vi "Dual Camera Control.vi"(7 "Calling VI Ref":refnum<vi>) -> ()   [LabVIEW 2016]
uses:
  Dual Camera Controls/Dual Camera - Simple Control.ctl
  <vilib>/Utility/miscctls.llb/LVPointTypeDef.ctl
  Hardware Configuration/Hardware Configuration Controls/Device Type.ctl
  Hardware Configuration/Hardware Configuration Controls/Device Function.ctl
  Device Library/Cameras/Photometrics/Prime BSI/Prime BSI Controls/Prime Actions.ctl
  Device Library/AOTF and AOM/AOTF Controls/AOTF Actions.ctl
  Device Library/Cameras/Photometrics/Prime BSI/Prime BSI Controls/Prime Parameters.ctl
  Device Library/Cameras/Photometrics/Prime BSI/Prime BSI Controls/Prime Parameter List.ctl
  Device Library/Stages/Stages Controls/Stage Actions.ctl
  Device Library/Cameras/Photometrics/Prime BSI/Prime BSI Controls/Prime ROI.ctl
  <vilib>/vision/Image Controls.llb/IMAQ Image.ctl
panel:
  in  "WFDC Z Step":bool
  in  "No. of Steps":i32
  in  "Step Size (µm)":dbl
  in  "Z Stack":bool
  in  "Cycles":u32
  in  "Delay Time (s)":u32
  in  "Delay Capture":bool
  in  "Both Cameras":T1 {"Exposure Time (s)" format="%#_4g"}
  in  "Camera 02":T1 {"Exposure Time (s)" format="%#_4g"}
  in  "Camera 01":T1 {"Exposure Time (s)" format="%#_4g"}
  in  "Quit":bool
  # "Camera 01"
  # "Camera 02"
  # "Both Cams"
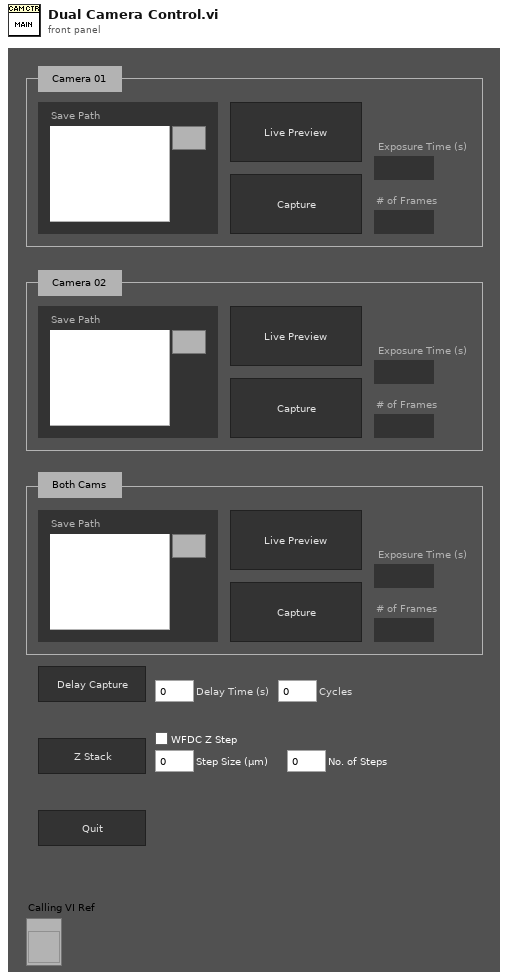
[diagram p1: front panel]
types:
  T1 = typedef "Dual Camera - Simple Control.ctl" = cluster{"Save Path":path, "Live Preview":bool, "Capture":bool, "Exposure Time (s)":dbl, "# of Frames":u32}
  T2 = enum16{"Always On", "Always Off", "Off While Running"}
  T3 = typedef "LVPointTypeDef.ctl" = cluster{"Horizontal":i16, "Vertical":i16}
  T4 = typedef "Device Function.ctl" = enum16{"Primary", "Secondary", "Overview", "Wide Field Drift Correction", "642 nm Excitation", "560 nm Excitation", "546 nm Excitation", "488 nm Excitation", "405 nm Excitation", "Objective Drift Correction", "Objective XY", "Objective Z", "Sample XY", "Sample Coarse Z", "Sample Z", "4Pi Lower", "4Pi Upper", "Adj Cavity", "Line Scanning", "Alert"}
  T5 = typedef "Device Type.ctl" = enum16{"AOTF", "Camera", "Deformable Mirror", "Laser", "Shutter", "Stage", "Waveform", "Email"}
  T6 = typedef "IMAQ Image.ctl" = refnum<image>
  T7 = typedef "Prime ROI.ctl" = cluster{"X Start":u32, "X End":u32, "X Bin":u32, "Y Start":u32, "Y End":u32, "Y Bin":u32}
  T8 = typedef "Prime Parameters.ctl" = cluster{"Parameter":T9, "Value":dbl}
  T9 = typedef "Prime Parameter List.ctl" = enum16{"Exposure Time (s)"}
  T10 = typedef "Prime Actions.ctl" = enum16{"Error Check", "Initialize", "Preview", "Record", "Abort", "Record Settings", "Set Parameter", "Get Parameter", "Set ROI", "Get ROI", "Status", "Set Trigger", "Quit"}
  T11 = typedef "AOTF Actions.ctl" = enum16{"Error Check", "Blank", "Line On/Off", "Set Power", "Status", "Quit"}
  T12 = typedef "Stage Actions.ctl" = enum16{"Get Position", "MVR", "MOVE", "HALT", "ONTARGET", "ERROR", "REFERENCE", "INIT", "VELOCITY", "STATUS", "EXIT", "HOME", "ZEROPOS", "NANOPOS", "ANALOG", "QUIT"}
  T13 = enum8{"Enabled", "Disabled", "Disabled and Grayed Out"}
  T14 = cluster{"Save Path":bool, "Live Preview":bool, "Capture":bool, "Exposure Time (s)":bool, "# of Frames":bool}
  T15 = typedef "LVRectTypeDef.ctl" = cluster{"Left":i16, "Top":i16, "Right":i16, "Bottom":i16}
  T16 = typedef "LVBoundsTypeDef.ctl" = cluster{"Width":u32, "Height":u32}
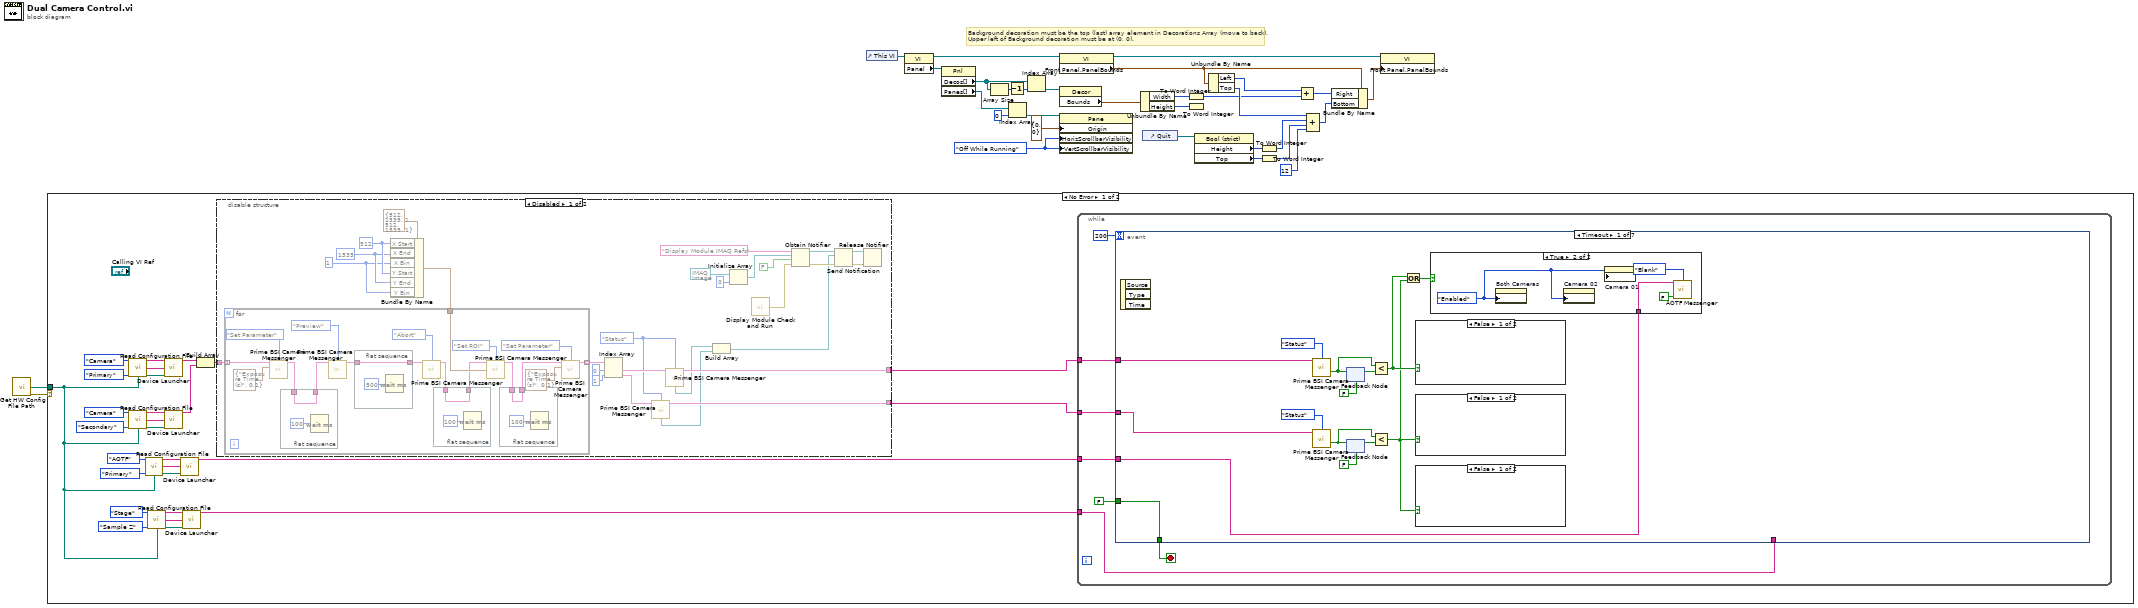
[diagram p0: block diagram]
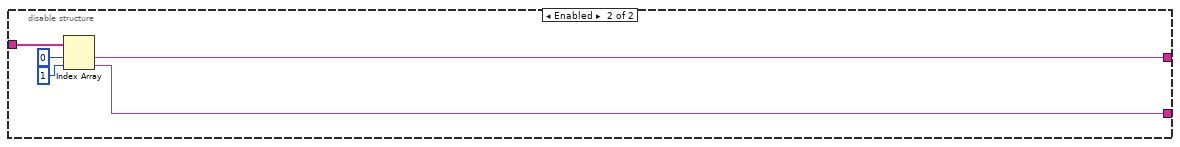
[diagram p2: hidden frame]
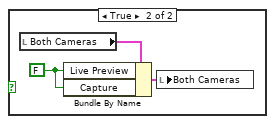
[diagram p4: hidden frame]
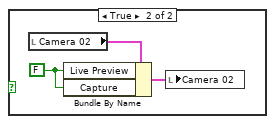
[diagram p5: hidden frame]
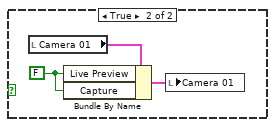
[diagram p6: hidden frame]
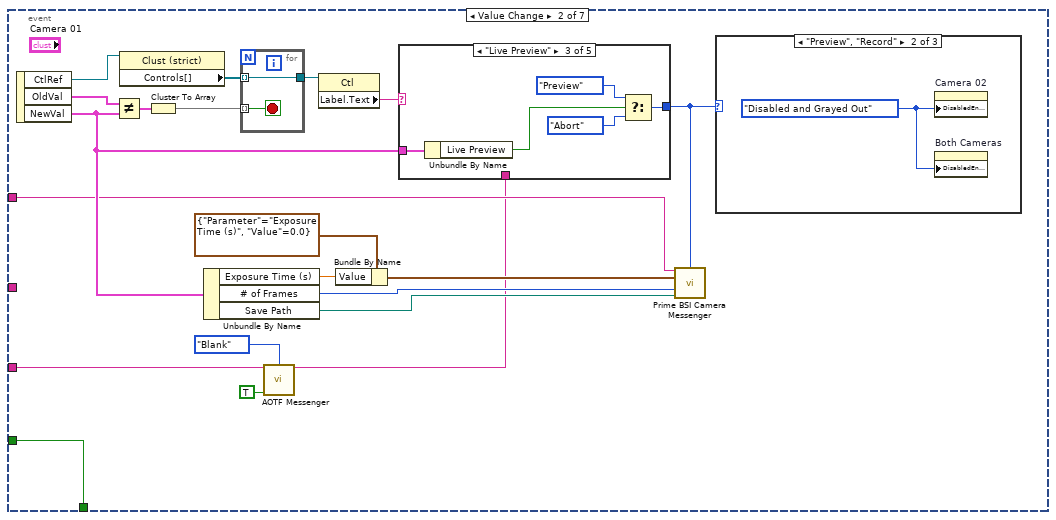
[diagram p7: hidden frame]
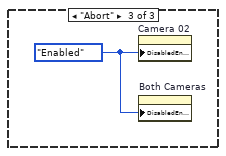
[diagram p9: hidden frame]
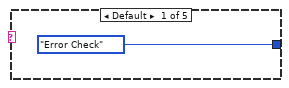
[diagram p10: hidden frame]
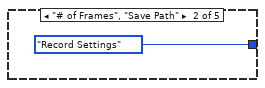
[diagram p11: hidden frame]
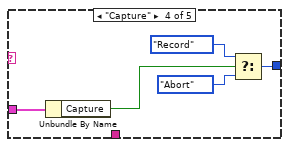
[diagram p12: hidden frame]
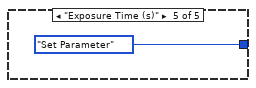
[diagram p13: hidden frame]
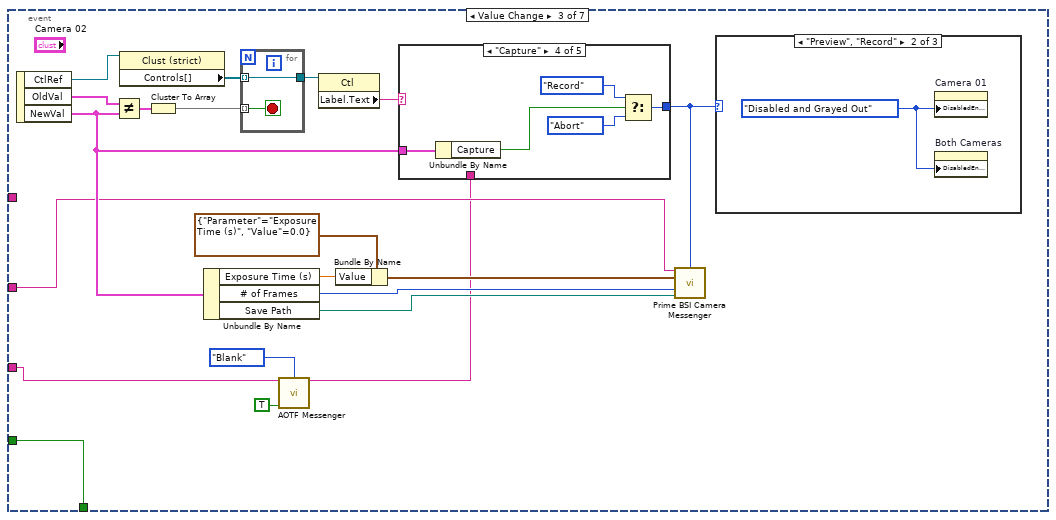
[diagram p14: hidden frame]
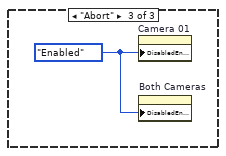
[diagram p16: hidden frame]
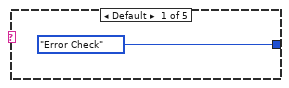
[diagram p17: hidden frame]
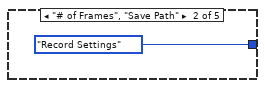
[diagram p18: hidden frame]
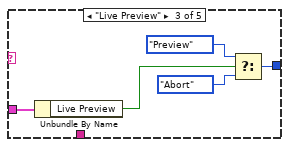
[diagram p19: hidden frame]
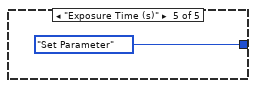
[diagram p20: hidden frame]
diagram:
  w14 = T2."Off While Running" ("Vertical Scrollbar Visibility")
  # "Background decoration must be the top (last) array element in Decorations Array (move to back).\nUpper left of Background decoration must be at (0, 0)."
  n1 = call "Get HW Config File Path.vi"() -> ("File Path"=w1:path, "Error"=w2:errorcluster)  [unwired: 14 in]
  n2 = case shown="No Error" w2 {
    tunnel: w1 -> [w38 _]
    frame No Error {
      n3 = call "Read Configuration File.vi"("Device Type"=Device_Type."Camera", "Device Function"=Device_Function."Primary", "Config File Path"=w38) -> ("Unique Notifier Name"=w59:string, "Device Ports/IDs/Channels"=w57:string[], "Device Engine Path"=w58:path)  [unwired: 9 in, 1 out]
      n4 = call "Read Configuration File.vi"("Device Type"=Device_Type."Camera", "Device Function"=Device_Function."Secondary", "Config File Path"=w38) -> ("Unique Notifier Name"=w50:string, "Device Ports/IDs/Channels"=w52:string[], "Device Engine Path"=w51:path)  [unwired: 9 in, 1 out]
      n5 = call "Read Configuration File.vi"("Device Type"=Device_Type."AOTF", "Device Function"=Device_Function."Primary", "Config File Path"=w38) -> ("Unique Notifier Name"=w49:string, "Device Ports/IDs/Channels"=w47:string[], "Device Engine Path"=w48:path)  [unwired: 9 in, 1 out]
      n6 = call "Read Configuration File.vi"("Device Type"=Device_Type."Stage", "Device Function"=Device_Function."Sample Z", "Config File Path"=w38) -> ("Unique Notifier Name"=w39:string, "Device Ports/IDs/Channels"=w41:string[], "Device Engine Path"=w40:path)  [unwired: 9 in, 1 out]
      n7 = call "Device Launcher.vi"("Notifier Name"=w59, "Device Ports/IDs/Channels"=w57, "Device Engine Path"=w58) -> ("Notifier Name"=w36:string)  [unwired: 11 in, 1 out]
      n8 = call "Device Launcher.vi"("Notifier Name"=w50, "Device Ports/IDs/Channels"=w52, "Device Engine Path"=w51) -> ("Notifier Name"=w35:string)  [unwired: 11 in, 1 out]
      n9 = call "Device Launcher.vi"("Notifier Name"=w49, "Device Ports/IDs/Channels"=w47, "Device Engine Path"=w48) -> ("Notifier Name"=w44:string)  [unwired: 11 in, 1 out]
      n10 = call "Device Launcher.vi"("Notifier Name"=w39, "Device Ports/IDs/Channels"=w41, "Device Engine Path"=w40) -> ("Notifier Name"=w37:string)  [unwired: 11 in, 1 out]
      n11 = Build Array(w36, w35) -> (w34:string[])
      n12 = disable-structure shown="Disabled" {
        disable-tunnel: w34 -> [w86 w115]
        disable-tunnel: [w76 w114] -> w33
        disable-tunnel: [w74 w113] -> w32
        frame Disabled {
          w75 = Prime_Actions."Status" ("Prime Actions")
          w79 = u32 1 ("X Bin")
          w80 = u32 1535 ("X End")
          w81 = u32 512 ("X Start")
          n13 = Bundle By Name(cluster=T7 {"X Start"=512, "X End"=1535, "X Bin"=1, "Y Start"=512, "Y End"=1535, "Y Bin"=1} ("ROI Setup"), "X Start"=w81, "X End"=w80, "X Bin"=w79, "Y Start"=w81, "Y End"=w80, "Y Bin"=w79) -> (w78:T7)
          n14 = for {
            tunnel: w86 -> [w95] mode=indexing
            tunnel: [w94] -> w85 mode=indexing
            tunnel: w78 -> [w93]
            n15 = call "Prime BSI Camera Messenger.vi"("Notifier Name"=w95, "Prime Actions"=Prime_Actions."Set Parameter", "Prime Parameter"=T8 {"Parameter"=enum."Exposure Time (s)", "Value"=0.1}) -> ("Notifier Name (Dup)"=w92:string)  [unwired: 7 in, 5 out]
            n16 = flat-sequence {
              tunnel: [w109] -> w91
              tunnel: w92 -> [w109]
              frame #0 {
                n17 = Wait (ms)(milliseconds to wait=u32 100) -> ()  [unwired: 1 out]
              }
            }
            n18 = call "Prime BSI Camera Messenger.vi"("Notifier Name"=w91, "Prime Actions"=Prime_Actions."Preview") -> ("Notifier Name (Dup)"=w102:string)  [unwired: 8 in, 5 out]
            n19 = flat-sequence {
              tunnel: w102 -> [w112]
              tunnel: [w112] -> w99
              frame #0 {
                n20 = Wait (ms)(milliseconds to wait=u32 500) -> ()  [unwired: 1 out]
              }
            }
            n21 = call "Prime BSI Camera Messenger.vi"("Notifier Name"=w99, "Prime Actions"=Prime_Actions."Abort") -> ("Notifier Name (Dup)"=w90:string)  [unwired: 8 in, 5 out]
            n22 = flat-sequence {
              tunnel: [w107] -> w89
              tunnel: w90 -> [w107]
              frame #0 {
                n23 = Wait (ms)(milliseconds to wait=u32 100) -> ()  [unwired: 1 out]
              }
            }
            n24 = call "Prime BSI Camera Messenger.vi"("Notifier Name"=w89, "Prime Actions"=Prime_Actions."Set ROI", "ROI Setup"=w93) -> ("Notifier Name (Dup)"=w88:string)  [unwired: 7 in, 5 out]
            n25 = flat-sequence {
              tunnel: [w105] -> w87
              tunnel: w88 -> [w105]
              frame #0 {
                n26 = Wait (ms)(milliseconds to wait=u32 100) -> ()  [unwired: 1 out]
              }
            }
            n27 = call "Prime BSI Camera Messenger.vi"("Notifier Name"=w87, "Prime Actions"=Prime_Actions."Set Parameter", "Prime Parameter"=T8 {"Parameter"=enum."Exposure Time (s)", "Value"=0.1}) -> ("Notifier Name (Dup)"=w94:string)  [unwired: 7 in, 5 out]
          }
          n28 = Index Array(array=w85, index #1=0 ("index"), index #2=1 ("index")) -> (element #1=w77:string, element #2=w60:string)
          n29 = call "Prime BSI Camera Messenger.vi"("Notifier Name"=w60, "Prime Actions"=w75) -> ("Notifier Name (Dup)"=w74:string, "Image Ref"=w72:T6)  [unwired: 8 in, 4 out]
          n30 = call "Prime BSI Camera Messenger.vi"("Notifier Name"=w77, "Prime Actions"=w75) -> ("Notifier Name (Dup)"=w76:string, "Image Ref"=w73:T6)  [unwired: 8 in, 4 out]
          n31 = Build Array(w73, w72) -> (w61:T6[])
          n32 = Initialize Array(T6 refnum ("New Image"), 0 ("dimension size")) -> (w70:T6[])
          n33 = call "Display Module Check and Run.vi"() -> ("Error"=w71:errorcluster)  [unwired: 15 in]
          n34 = Obtain Notifier(name (unnamed)="Display Module IMAQ Refs", notification data type=w70, create if not found? (T)=FALSE, error in (no error)=w71) -> (notifier out=w62:refnum<notifier>, error out=w65:errorcluster)  [unwired: 1 out]
          n35 = Send Notification(notification=w61, notifier=w62, error in (no error)=w65) -> (notifier out=w63:refnum<notifier>, error out=w64:errorcluster)
          n36 = Release Notifier(notifier=w63, error in (no error)=w64) -> ()  [unwired: 1 in, 3 out]
        }
        frame Enabled {
          n37 = Index Array(array=w115, index #1=0 ("index"), index #2=1 ("index")) -> (element #1=w114:string, element #2=w113:string)
        }
      }
      n38 = while {
        tunnel: w33 -> [w121]
        tunnel: w32 -> [w120]
        tunnel: w44 -> [w119]
        tunnel: w37 -> [w118]
        stop <- w123 stop-if-true
        n39 = event shown="[0] Timeout" {
          selector: _ -> [_ _ _ _ _ _ _]
          dyn-events: _ -> [_ _ _ _ _ _ _]
          timeout: 200 -> [_ _ _ _ _ _ _]
          tunnel: [w139 w172 w209 w255 w277 w349 w408] -> w123
          tunnel: FALSE -> [w139 w172 w209 w255 w277 w349 _]
          tunnel: w121 -> [w138 w158 _ w244 w276 w348 w407]
          tunnel: w120 -> [w129 _ w195 w241 w275 w347 w406]
          tunnel: w119 -> [w125 w156 w191 w228 w274 w344 _]
          tunnel: w118 -> [_ _ _ _ _ w333 _]
          event Timeout {
            n40 = event-data() -> ()  [unwired: 1 in, 3 out]
            n41 = call "Prime BSI Camera Messenger.vi"("Notifier Name"=w138, "Prime Actions"=Prime_Actions."Status") -> ("Running?"=w134:bool)  [unwired: 8 in, 5 out]
            n42 = call "Prime BSI Camera Messenger.vi"("Notifier Name"=w129, "Prime Actions"=Prime_Actions."Status") -> ("Running?"=w130:bool)  [unwired: 8 in, 5 out]
            n43 = feedback-in #1(w134) -> ()
            n44 = feedback #1(FALSE) -> (w135:bool)
            n45 = feedback #2(FALSE) -> (w131:bool)
            n46 = feedback-in #2(w130) -> ()
            n47 = Less?(x=w134, y=w135) -> (x < y?=w128:bool)
            n48 = Less?(x=w130, y=w131) -> (x < y?=w127:bool)
            n49 = Or(x=w128, y=w127) -> (x .or. y?=w126:bool)
            n50 = case shown="False" w128 {
              frame False {
              }
              frame True {
                w151 = FALSE ("Live Preview")
                n51 = local read "Camera 01"() -> (w152:T1)
                n52 = Bundle By Name(cluster=w152, "Live Preview"=w151, "Capture"=w151) -> (w150:T1)
                n53 = local write "Camera 01"(w150) -> ()
              }
            }
            n54 = case shown="False" w127 {
              frame False {
              }
              frame True {
                w148 = FALSE ("Live Preview")
                n55 = local read "Camera 02"() -> (w149:T1)
                n56 = Bundle By Name(cluster=w149, "Live Preview"=w148, "Capture"=w148) -> (w147:T1)
                n57 = local write "Camera 02"(w147) -> ()
              }
            }
            n58 = case shown="False" w127 {
              frame False {
              }
              frame True {
                w145 = FALSE ("Live Preview")
                n59 = local read "Both Cameras"() -> (w146:T1)
                n60 = Bundle By Name(cluster=w146, "Live Preview"=w145, "Capture"=w145) -> (w144:T1)
                n61 = local write "Both Cameras"(w144) -> ()
              }
            }
            n62 = case shown="True" w126 {
              tunnel: w125 -> [_ w140]
              frame False {
              }
              frame True {
                w143 = T13."Enabled" ("Disabled")
                n63 = property on="Both Cameras" class="Clust (strict)"("DisabledEnum"=w143) -> ()  [unwired: 2 in, 2 out]
                n64 = property on="Camera 02" class="Clust (strict)"("DisabledEnum"=w143) -> ()  [unwired: 2 in, 2 out]
                n65 = property on="Camera 01" class="Clust (strict)"("DisabledEnum"=w143) -> ()  [unwired: 2 in, 2 out]
                n66 = call "AOTF Messenger.vi"("AOTF Notifier Name"=w140, "AOTF Action"=AOTF_Actions."Blank", "Beam Blank"=FALSE) -> ()  [unwired: 8 in, 5 out]
              }
            }
          }
          event Value Change {
            n67 = event-data() -> ("CtlRef"=w170:refnum<vi>, "OldVal"=w171:T1, "NewVal"=w159:T1)  [unwired: 1 in]
            n68 = Not Equal?(x=w171, y=w159) -> (x != y?=w169:T14)
            n69 = property class="Clust (strict)"(reference=w170) -> ("Controls[]"=w167:refnum<vi>[])  [unwired: 1 in, 2 out]
            n70 = Cluster To Array(cluster=w169) -> (array=w168:bool[])
            n71 = Unbundle By Name(w159) -> ("Exposure Time (s)"=w161:dbl, "# of Frames"=w163:u32, "Save Path"=w164:path)
            n72 = for {
              tunnel: w168 -> [w189] mode=indexing
              tunnel: w167 -> [w188] mode=indexing
              tunnel: [w188] -> w166
              stop <- w189 stop-if-true
            }
            n73 = call "AOTF Messenger.vi"("AOTF Notifier Name"=w156, "AOTF Action"=AOTF_Actions."Blank", "Beam Blank"=TRUE) -> ("AOTF Notifier Name (Dup)"=w153:string)  [unwired: 8 in, 4 out]
            n74 = property class="Ctl"(reference=w166) -> ("Label.Text"=w165:string)  [unwired: 1 in, 2 out]
            n75 = Bundle By Name(cluster=T8 {"Parameter"=enum."Exposure Time (s)", "Value"=0.0} ("Prime Parameter"), "Value"=w161) -> (w160:T8)
            n76 = case shown="\"Live Preview\"" w165 {
              tunnel: [Prime_Actions."Error Check" ("Prime Actions") Prime_Actions."Record Settings" ("Prime Actions") w179 w184 Prime_Actions."Set Parameter" ("Prime Actions")] -> w157
              tunnel: w159 -> [_ _ w178 w183 _]
              tunnel: w153 -> [_ _ _ _ _]
              frame Default {
              }
              frame "# of Frames", "Save Path" {
              }
              frame "Live Preview" {
                n77 = Unbundle By Name(w178) -> ("Live Preview"=w177:bool)
                n78 = Select(t=Prime_Actions."Preview" ("Prime Actions"), s=w177, f=Prime_Actions."Abort") -> (s? t:f=w179:T10)
              }
              frame "Capture" {
                n79 = Unbundle By Name(w183) -> ("Capture"=w182:bool)
                n80 = Select(t=Prime_Actions."Record" ("Prime Actions"), s=w182, f=Prime_Actions."Abort") -> (s? t:f=w184:T10)
              }
              frame "Exposure Time (s)" {
              }
            }
            n81 = call "Prime BSI Camera Messenger.vi"("Notifier Name"=w158, "Prime Actions"=w157, "Prime Parameter"=w160, "# of Frames"=w163, "File Save Path"=w164) -> ()  [unwired: 5 in, 6 out]
            n82 = case shown="\"Preview\", \"Record\"" w157 {
              frame Default {
              }
              frame "Preview", "Record" {
                w173 = T13."Disabled and Grayed Out" ("Disabled")
                n83 = property on="Camera 02" class="Clust (strict)"("DisabledEnum"=w173) -> ()  [unwired: 2 in, 2 out]
                n84 = property on="Both Cameras" class="Clust (strict)"("DisabledEnum"=w173) -> ()  [unwired: 2 in, 2 out]
              }
              frame "Abort" {
                w174 = T13."Enabled" ("Disabled")
                n85 = property on="Camera 02" class="Clust (strict)"("DisabledEnum"=w174) -> ()  [unwired: 2 in, 2 out]
                n86 = property on="Both Cameras" class="Clust (strict)"("DisabledEnum"=w174) -> ()  [unwired: 2 in, 2 out]
              }
            }
          }
          event Value Change {
            n87 = event-data() -> ("CtlRef"=w207:refnum<vi>, "OldVal"=w208:T1, "NewVal"=w196:T1)  [unwired: 1 in]
            n88 = Not Equal?(x=w208, y=w196) -> (x != y?=w206:T14)
            n89 = property class="Clust (strict)"(reference=w207) -> ("Controls[]"=w204:refnum<vi>[])  [unwired: 1 in, 2 out]
            n90 = Cluster To Array(cluster=w206) -> (array=w205:bool[])
            n91 = Unbundle By Name(w196) -> ("Exposure Time (s)"=w198:dbl, "# of Frames"=w200:u32, "Save Path"=w201:path)
            n92 = for {
              tunnel: w205 -> [w226] mode=indexing
              tunnel: w204 -> [w225] mode=indexing
              tunnel: [w225] -> w203
              stop <- w226 stop-if-true
            }
            n93 = call "AOTF Messenger.vi"("AOTF Notifier Name"=w191, "AOTF Action"=AOTF_Actions."Blank", "Beam Blank"=TRUE) -> ("AOTF Notifier Name (Dup)"=w190:string)  [unwired: 8 in, 4 out]
            n94 = property class="Ctl"(reference=w203) -> ("Label.Text"=w202:string)  [unwired: 1 in, 2 out]
            n95 = Bundle By Name(cluster=T8 {"Parameter"=enum."Exposure Time (s)", "Value"=0.0} ("Prime Parameter"), "Value"=w198) -> (w197:T8)
            n96 = case shown="\"Capture\"" w202 {
              tunnel: [Prime_Actions."Error Check" ("Prime Actions") Prime_Actions."Record Settings" ("Prime Actions") w216 w221 Prime_Actions."Set Parameter" ("Prime Actions")] -> w194
              tunnel: w196 -> [_ _ w215 w220 _]
              tunnel: w190 -> [_ _ _ _ _]
              frame Default {
              }
              frame "# of Frames", "Save Path" {
              }
              frame "Live Preview" {
                n97 = Unbundle By Name(w215) -> ("Live Preview"=w214:bool)
                n98 = Select(t=Prime_Actions."Preview" ("Prime Actions"), s=w214, f=Prime_Actions."Abort") -> (s? t:f=w216:T10)
              }
              frame "Capture" {
                n99 = Unbundle By Name(w220) -> ("Capture"=w219:bool)
                n100 = Select(t=Prime_Actions."Record" ("Prime Actions"), s=w219, f=Prime_Actions."Abort") -> (s? t:f=w221:T10)
              }
              frame "Exposure Time (s)" {
              }
            }
            n101 = call "Prime BSI Camera Messenger.vi"("Notifier Name"=w195, "Prime Actions"=w194, "Prime Parameter"=w197, "# of Frames"=w200, "File Save Path"=w201) -> ()  [unwired: 5 in, 6 out]
            n102 = case shown="\"Preview\", \"Record\"" w194 {
              frame Default {
              }
              frame "Preview", "Record" {
                w210 = T13."Disabled and Grayed Out" ("Disabled")
                n103 = property on="Camera 01" class="Clust (strict)"("DisabledEnum"=w210) -> ()  [unwired: 2 in, 2 out]
                n104 = property on="Both Cameras" class="Clust (strict)"("DisabledEnum"=w210) -> ()  [unwired: 2 in, 2 out]
              }
              frame "Abort" {
                w211 = T13."Enabled" ("Disabled")
                n105 = property on="Camera 01" class="Clust (strict)"("DisabledEnum"=w211) -> ()  [unwired: 2 in, 2 out]
                n106 = property on="Both Cameras" class="Clust (strict)"("DisabledEnum"=w211) -> ()  [unwired: 2 in, 2 out]
              }
            }
          }
          event Value Change {
            n107 = event-data() -> ("CtlRef"=w253:refnum<vi>, "OldVal"=w254:T1, "NewVal"=w245:T1)  [unwired: 1 in]
            n108 = Not Equal?(x=w254, y=w245) -> (x != y?=w252:T14)
            n109 = property class="Clust (strict)"(reference=w253) -> ("Controls[]"=w250:refnum<vi>[])  [unwired: 1 in, 2 out]
            n110 = Cluster To Array(cluster=w252) -> (array=w251:bool[])
            n111 = Unbundle By Name(w245) -> ("Exposure Time (s)"=w246:dbl, "# of Frames"=w243:u32, "Save Path"=w240:path)
            n112 = call "AOTF Messenger.vi"("AOTF Notifier Name"=w228, "AOTF Action"=AOTF_Actions."Blank", "Beam Blank"=TRUE) -> ("AOTF Notifier Name (Dup)"=w227:string)  [unwired: 8 in, 4 out]
            n113 = for {
              tunnel: w251 -> [w272] mode=indexing
              tunnel: w250 -> [w271] mode=indexing
              tunnel: [w271] -> w249
              stop <- w272 stop-if-true
            }
            n114 = property class="Ctl"(reference=w249) -> ("Label.Text"=w248:string)  [unwired: 1 in, 2 out]
            n115 = Bundle By Name(cluster=T8 {"Parameter"=enum."Exposure Time (s)", "Value"=0.0} ("Prime Parameter"), "Value"=w246) -> (w242:T8)
            n116 = Strip Path(path=w240) -> (stripped path=w234:path, name=w232:string)
            n117 = case shown="\"# of Frames\", \"Save Path\"" w248 {
              tunnel: [Prime_Actions."Error Check" ("Prime Actions") Prime_Actions."Record Settings" ("Prime Actions") w262 w267 Prime_Actions."Set Parameter" ("Prime Actions")] -> w231
              tunnel: w245 -> [_ _ w261 w266 _]
              tunnel: w227 -> [_ _ _ _ _]
              frame Default {
              }
              frame "# of Frames", "Save Path" {
              }
              frame "Live Preview" {
                n118 = Unbundle By Name(w261) -> ("Live Preview"=w260:bool)
                n119 = Select(t=Prime_Actions."Preview" ("Prime Actions"), s=w260, f=Prime_Actions."Abort") -> (s? t:f=w262:T10)
              }
              frame "Capture" {
                n120 = Unbundle By Name(w266) -> ("Capture"=w265:bool)
                n121 = Select(t=Prime_Actions."Record" ("Prime Actions"), s=w265, f=Prime_Actions."Abort") -> (s? t:f=w267:T10)
              }
              frame "Exposure Time (s)" {
              }
            }
            n122 = Concatenate Strings(w232, " - Camera 01" ("string")) -> (w235:string)
            n123 = Concatenate Strings(w232, " - Camera 02" ("string")) -> (w238:string)
            n124 = Build Path(base path=w234, name or relative path=w235) -> (appended path=w233:path)
            n125 = Build Path(base path=w234, name or relative path=w238) -> (appended path=w237:path)
            n126 = call "Prime BSI Camera Messenger.vi"("Notifier Name"=w244, "Prime Actions"=w231, "Prime Parameter"=w242, "# of Frames"=w243, "File Save Path"=w233) -> ()  [unwired: 5 in, 6 out]
            n127 = call "Prime BSI Camera Messenger.vi"("Notifier Name"=w241, "Prime Actions"=w231, "Prime Parameter"=w242, "# of Frames"=w243, "File Save Path"=w237) -> ()  [unwired: 5 in, 6 out]
            n128 = case shown="\"Abort\"" w231 {
              frame Default {
              }
              frame "Preview", "Record" {
                w256 = T13."Disabled and Grayed Out" ("Disabled")
                n129 = property on="Camera 01" class="Clust (strict)"("DisabledEnum"=w256) -> ()  [unwired: 2 in, 2 out]
                n130 = property on="Camera 02" class="Clust (strict)"("DisabledEnum"=w256) -> ()  [unwired: 2 in, 2 out]
              }
              frame "Abort" {
                w257 = T13."Enabled" ("Disabled")
                n131 = property on="Camera 01" class="Clust (strict)"("DisabledEnum"=w257) -> ()  [unwired: 2 in, 2 out]
                n132 = property on="Camera 02" class="Clust (strict)"("DisabledEnum"=w257) -> ()  [unwired: 2 in, 2 out]
              }
            }
          }
          event "Delay Capture": Value Change {
            n133 = event-data() -> ()  [unwired: 1 in, 3 out]
            n134 = while {
              tunnel: w276 -> [w291]
              tunnel: w275 -> [w290]
              tunnel: w274 -> [w289]
              tunnel: [FALSE ("Delay Capture")] -> w273
              i -> [w288]
              stop <- w278 stop-if-true
              n135 = flat-sequence {
                tunnel: w290 -> [w300]
                tunnel: w291 -> [w301]
                tunnel: [w301] -> w295
                tunnel: [w300] -> w294
                tunnel: w289 -> [w297]
                tunnel: [w296] -> w293
                tunnel: w295 -> [w318]
                tunnel: w294 -> [w316]
                tunnel: w293 -> [w303]
                tunnel: [w303] -> w292
                tunnel: [w302] -> w280
                tunnel: w292 -> [w321]
                tunnel: [w321] -> w281
                tunnel: w280 -> [w320]
                tunnel: w281 -> [w327]
                tunnel: w278 -> [w326]
                frame #0 {
                  n136 = call "AOTF Messenger.vi"("AOTF Notifier Name"=w297, "AOTF Action"=AOTF_Actions."Blank", "Beam Blank"=TRUE) -> ("AOTF Notifier Name (Dup)"=w296:string)  [unwired: 8 in, 4 out]
                }
                frame #1 {
                  w304 = Prime_Actions."Record" ("Prime Actions")
                  n137 = local read "Both Cameras"() -> (w305:T1)
                  n138 = Unbundle By Name(w305) -> ("Exposure Time (s)"=w307:dbl, "Save Path"=w306:path)  [unwired: 1 out]
                  n139 = Bundle By Name(cluster=T8 {"Parameter"=enum."Exposure Time (s)", "Value"=0.0} ("Prime Parameter"), "Value"=w307) -> (w317:T8)
                  n140 = Strip Path(path=w306) -> (stripped path=w310:path, name=w308:string)
                  n141 = Concatenate Strings(w308, " - Camera 01" ("string")) -> (w311:string)
                  n142 = Concatenate Strings(w308, " - Camera 02" ("string")) -> (w314:string)
                  n143 = Build Path(base path=w310, name or relative path=w311) -> (appended path=w309:path)
                  n144 = Build Path(base path=w310, name or relative path=w314) -> (appended path=w313:path)
                  n145 = call "Prime BSI Camera Messenger.vi"("Notifier Name"=w318, "Prime Actions"=w304, "Prime Parameter"=w317, "File Save Path"=w309) -> ("Notifier Name (Dup)"=w302:string)  [unwired: 6 in, 5 out]
                  n146 = call "Prime BSI Camera Messenger.vi"("Notifier Name"=w316, "Prime Actions"=w304, "Prime Parameter"=w317, "File Save Path"=w313) -> ()  [unwired: 6 in, 6 out]
                }
                frame #2 {
                  n147 = while {
                    tunnel: w320 -> [w325]
                    stop <- w323 continue-if-true
                    n148 = call "Prime BSI Camera Messenger.vi"("Notifier Name"=w325, "Prime Actions"=Prime_Actions."Status") -> ("Running?"=w323:bool)  [unwired: 8 in, 5 out]
                    n149 = Wait (ms)(milliseconds to wait=u32 5) -> ()  [unwired: 1 out]
                  }
                }
                frame #3 {
                  n150 = case shown="False" w326 {
                    frame False {
                      n151 = Multiply(x="Delay Time (s)", y=u32 1000) -> (x*y=w330:u32)
                      n152 = Wait (ms)(milliseconds to wait=w330) -> ()  [unwired: 1 out]
                    }
                    frame True {
                    }
                  }
                  n153 = call "AOTF Messenger.vi"("AOTF Notifier Name"=w327, "AOTF Action"=AOTF_Actions."Blank", "Beam Blank"=FALSE) -> ()  [unwired: 8 in, 5 out]
                }
              }
              n154 = To Unsigned Long Integer(number=w288) -> (unsigned 32bit integer=w285:u32)
              n155 = Increment(x=w285) -> (x+1=w287:u32)
              n156 = Greater Or Equal?(x=w287, y="Cycles") -> (x >= y?=w284:bool)
              n157 = Not(x="Delay Capture") -> (.not. x?=w282:bool)
              n158 = Or(x=w284, y=w282) -> (x .or. y?=w278:bool)
            }
            n159 = property on="Delay Capture" class="Bool (strict)"("Value"=w273) -> ()  [unwired: 2 in, 2 out]
          }
          event "Z Stack": Value Change {
            w336 = 0.0
            n160 = event-data() -> ()  [unwired: 1 in, 3 out]
            n161 = call "AOTF Messenger.vi"("AOTF Notifier Name"=w344, "AOTF Action"=AOTF_Actions."Blank", "Beam Blank"=TRUE) -> ("AOTF Notifier Name (Dup)"=w343:string)  [unwired: 8 in, 4 out]
            n162 = Obtain Notifier(name (unnamed)="WFDC Z Step", notification data type=w336) -> (notifier out=w337:refnum<notifier>)  [unwired: 2 in, 2 out]
            n163 = Send Notification(notification=w336, notifier=w337) -> (notifier out=w335:refnum<notifier>)  [unwired: 1 in, 1 out]
            n164 = while {
              tunnel: w348 -> [w360]
              tunnel: w347 -> [w359]
              tunnel: w343 -> [w357]
              tunnel: [w357] -> w340
              tunnel: "No. of Steps" -> [w356]
              tunnel: w335 -> [w353]
              tunnel: [FALSE] -> w334
              tunnel: w333 -> [w350]
              i -> [w355]
              stop <- w352 stop-if-true
              n165 = Increment(x=w355) -> (x+1=w354:i32)
              n166 = flat-sequence {
                tunnel: [w361] -> w358
                tunnel: w360 -> [w376]
                tunnel: w359 -> [w374]
                tunnel: w358 -> [w378]
                tunnel: w353 -> [w387]
                tunnel: w352 -> [w386]
                tunnel: w350 -> [w384]
                frame #0 {
                  w362 = Prime_Actions."Record" ("Prime Actions")
                  n167 = local read "Both Cameras"() -> (w363:T1)
                  n168 = Unbundle By Name(w363) -> ("Exposure Time (s)"=w365:dbl, "Save Path"=w364:path)  [unwired: 1 out]
                  n169 = Bundle By Name(cluster=T8 {"Parameter"=enum."Exposure Time (s)", "Value"=0.0} ("Prime Parameter"), "Value"=w365) -> (w375:T8)
                  n170 = Strip Path(path=w364) -> (stripped path=w368:path, name=w366:string)
                  n171 = Concatenate Strings(w366, " - Camera 01" ("string")) -> (w369:string)
                  n172 = Concatenate Strings(w366, " - Camera 02" ("string")) -> (w372:string)
                  n173 = Build Path(base path=w368, name or relative path=w369) -> (appended path=w367:path)
                  n174 = Build Path(base path=w368, name or relative path=w372) -> (appended path=w371:path)
                  n175 = call "Prime BSI Camera Messenger.vi"("Notifier Name"=w376, "Prime Actions"=w362, "Prime Parameter"=w375, "File Save Path"=w367) -> ("Notifier Name (Dup)"=w361:string)  [unwired: 6 in, 5 out]
                  n176 = call "Prime BSI Camera Messenger.vi"("Notifier Name"=w374, "Prime Actions"=w362, "Prime Parameter"=w375, "File Save Path"=w371) -> ()  [unwired: 6 in, 6 out]
                }
                frame #1 {
                  n177 = while {
                    tunnel: w378 -> [w382]
                    stop <- w380 continue-if-true
                    n178 = call "Prime BSI Camera Messenger.vi"("Notifier Name"=w382, "Prime Actions"=Prime_Actions."Status") -> ("Running?"=w380:bool)  [unwired: 8 in, 5 out]
                    n179 = Wait (ms)(milliseconds to wait=u32 5) -> ()  [unwired: 1 out]
                  }
                }
                frame #2 {
                  n180 = case shown="False" "WFDC Z Step" {
                    tunnel: w387 -> [_ w398]
                    tunnel: w386 -> [_ w395]
                    tunnel: w384 -> [w393 _]
                    tunnel: "Step Size (µm)" -> [w392 w394]
                    frame False {
                      n181 = Build Array(w392) -> (w391:dbl[])
                      n182 = Build Array(TRUE) -> (w389:bool[])
                      n183 = call "Stages Messenger.vi"("Stage Notifier Name"=w393, "Actions"=Stage_Actions."MVR", "Setpoint"=w391, "Axis"=w389) -> ()  [unwired: 8 in, 4 out]
                    }
                    frame True {
                      n184 = case shown="False" w395 {
                        tunnel: w398 -> [w403 w405]
                        tunnel: [w402 w405] -> w397
                        tunnel: [w400 0.0] -> w396
                        tunnel: w394 -> [w399 _]
                        frame False {
                          n185 = Get Notifier Status(notifier=w403) -> (notifier out=w402:refnum<notifier>, current notification=w401:dbl)  [unwired: 1 in, 3 out]
                          n186 = Add(x=w401, y=w399) -> (x+y=w400:dbl)
                        }
                        frame True {
                        }
                      }
                      n187 = Send Notification(notification=w396, notifier=w397) -> ()  [unwired: 1 in, 2 out]
                    }
                  }
                }
              }
              n188 = Equal?(x=w356, y=w354) -> (x = y?=w352:bool)
            }
            n189 = call "AOTF Messenger.vi"("AOTF Notifier Name"=w340, "AOTF Action"=AOTF_Actions."Blank", "Beam Blank"=FALSE) -> ()  [unwired: 8 in, 5 out]
            n190 = property on="Z Stack" class="Bool (strict)"("Value"=w334) -> ()  [unwired: 2 in, 2 out]
          }
          event "Quit": Value Change {
            n191 = event-data() -> ("NewVal"=w408:bool)  [unwired: 1 in]
            n192 = disable-structure shown="Enabled" {
              disable-tunnel: w407 -> [w412 _]
              disable-tunnel: w406 -> [w409 _]
              frame Disabled {
                n193 = call "Prime BSI Camera Messenger.vi"("Notifier Name"=w412, "Prime Actions"=Prime_Actions."Quit") -> ()  [unwired: 8 in, 6 out]
                n194 = call "Prime BSI Camera Messenger.vi"("Notifier Name"=w409, "Prime Actions"=Prime_Actions."Quit") -> ()  [unwired: 8 in, 6 out]
              }
              frame Enabled {
              }
            }
          }
        }
      }
    }
    frame Error {
    }
  }
  n195 = control-ref of="This VI"() -> (w6:refnum<vi>)
  n196 = property class="VI"(reference=w6) -> (reference out=w15:refnum<vi>, "Panel"=w7:refnum<vi>)  [unwired: 1 in, 1 out]
  n197 = property class="Pnl"(reference=w7) -> ("Decos[]"=w5:refnum<vi>[], "Panes[]"=w11:refnum<vi>[])  [unwired: 1 in, 2 out]
  n198 = Array Size(array=w5) -> (size(s)=w3:i32)
  n199 = Decrement(x=w3) -> (x-1=w4:i32)
  n200 = Index Array(array=w11, index=0) -> (element=w10:refnum<vi>)
  n201 = Index Array(array=w5, index=w4) -> (element=w13:refnum<vi>)
  n202 = property class="VI"(reference=w15) -> (reference out=w17:refnum<vi>, "Front Panel.PanelBounds"=w18:T15)  [unwired: 1 in, 1 out]
  n203 = property class="Decor"(reference=w13) -> ("Bounds"=w16:T16)  [unwired: 1 in, 2 out]
  n204 = property class="Pane"(reference=w10, "Origin"=T3 {"Horizontal"=0, "Vertical"=0}, "HorizScrollbarVisibility"=w14, "VertScrollbarVisibility"=w14) -> ()  [unwired: 1 in, 2 out]
  n205 = Unbundle By Name(w16) -> ("Width"=w21:u32, "Height"=w24:u32)
  n206 = control-ref of="Quit"() -> (w8:refnum<vi>)
  n207 = To Word Integer(number=w21) -> (16bit integer=w23:i16)
  n208 = To Word Integer(number=w24) -> ()  [unwired: 1 out]
  n209 = property class="Bool (strict)"(reference=w8) -> ("Height"=w26:u32, "Top"=w27:i32)  [unwired: 1 in, 2 out]
  n210 = Unbundle By Name(w18) -> ("Left"=w20:i16, "Top"=w31:i16)
  n211 = To Word Integer(number=w26) -> (16bit integer=w29:i16)
  n212 = To Word Integer(number=w27) -> (16bit integer=w30:i16)
  n213 = Add(x=w20, y=w23) -> (x+y=w22:i16)
  n214 = Compound Arithmetic op=ADD(w31, w29, w30, i16 12 ("y")) -> (w25:i16)
  n215 = Bundle By Name(cluster=w18, "Right"=w22, "Bottom"=w25) -> (w19:T15)
  n216 = property class="VI"(reference=w17, "Front Panel.PanelBounds"=w19) -> ()  [unwired: 1 in, 2 out]
